vi "Connect.vi"(8 "error in":errorcluster, 11 "2525 in":refnum<class "2525.lvclass">) -> (0 "error out":errorcluster, 3 "2525 out":refnum<class "2525.lvclass">)   [LabVIEW 2019, in "2525.lvlib" / "2525.lvclass"]
uses:
  Library/2525.lvclass
  C:/Users/Public/Documents/Development/builds/Instruments/Instruments.lvlibp/Library/Instruments.lvclass
  C:/Users/Public/Documents/Development/builds/Instruments/SwitchMatrix.lvlibp/Library/SwitchMatrix.lvclass
  Library/2525.lvclass/2525.ctl
  builds/Instruments/Instruments.lvlibp/Accessors/Read Simulated.vi
  builds/Instruments/Instruments.lvlibp/Accessors/Read Resource.vi
  builds/Instruments/SwitchMatrix.lvlibp/Accessors/Read Matrix Topology.vi
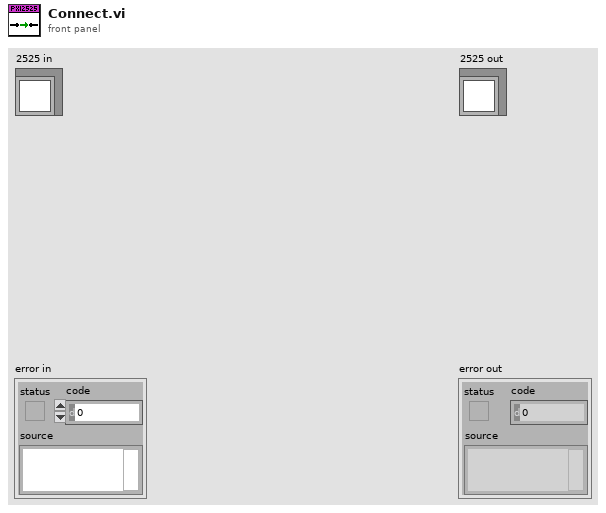
[diagram p1: front panel]
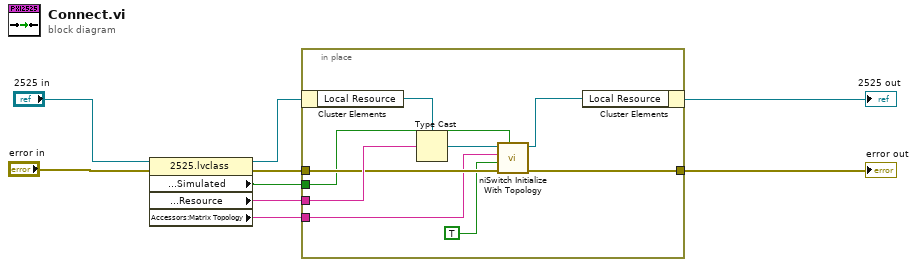
[diagram p0: block diagram]
diagram:
  n1 = property class="2525.lvclass"(reference="2525 in", error in="error in") -> (reference out=w6:refnum<class "2525.lvclass">, error out=w1:errorcluster, "Accessors:Configuration:Simulated"=w5:bool, "Accessors:Configuration:Resource"=w4:string, "Accessors:Matrix Topology"=w3:string)
  n2 = in-place {
    in-place-border: w4 -> [w17]
    in-place-border: [w14] -> w7
    in-place-border: w1 -> [w13]
    in-place-border: w5 -> [w11]
    in-place-border: w3 -> [w10]
    n3 = in-place-cluster #1(w6) -> ("Local Resource"=w16:refnum<k15>)
    n4 = Type Cast(type=w16, x=w17) -> (*(type *) &x=w18:refnum<k15>)
    n5 = call <instrlib>:"niSwitch Initialize With Topology.vi"("simulate (boolean value)"=w11, "error in (no error)"=w13, "reset device (boolean value)"=TRUE, "topology name"=w10, "resource name"=w18) -> ("error out"=w14:errorcluster, "instrument handle out"=w15:refnum<k15>)  [unwired: 5 in]
    n6 = in-place-cluster #1("Local Resource"=w15) -> (→"2525 out":refnum<class "2525.lvclass">)
  }
  "error out" <- w7
